vi "Write Pulse Recorder Configuration.vi"(8 "error in (no error)":errorcluster, 10 "Configuration":T1={"Pre-trigger duration"=0.01, "Post-trigger duration"=0.1, "Rate"=1000000.0, "Ranges"=[10.0], "Re-name channels"=[], "Active channels"="0:1", "External clock"=FALSE} {"Rate" format="%#_8pHz"; "Post-trigger duration" format="%#_6ps"; "Pre-trigger duration" format="%#_6ps"; "Ranges" format="%#_6pV"}, 11 "Pulse Recorder in":refnum<class "Pulse Recorder.lvclass">) -> (0 "error out":errorcluster, 3 "Pulse Recorder out":refnum<class "Pulse Recorder.lvclass">)   [LabVIEW 2016, in "Pulse Recorder.lvclass"]
uses:
  Pulse Recorder.lvclass
  C:/github/LabActor/Template Module/Template Module.lvclass
  NHMFL_Core/Libraries/Instruments/Pulse Driver/Pusle Driver Configuration.ctl
  Template Module/Template Module.lvclass/Template Module.ctl
  Template Module/Write Configuration.vi
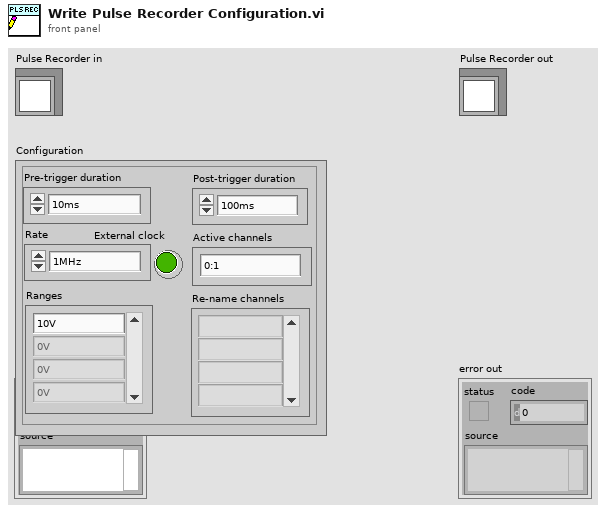
[diagram p1: front panel]
types:
  T1 = typedef "Pusle Driver Configuration.ctl" = cluster{"Pre-trigger duration":dbl, "Post-trigger duration":dbl, "Rate":dbl, "Ranges":dbl[], "Re-name channels":string[], "Active channels":string, "External clock":bool}
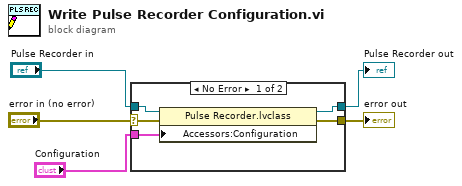
[diagram p0: block diagram]
diagram:
  n1 = case shown="No Error" "error in (no error)" {
    selector: "error in (no error)" -> [w7 w11]
    tunnel: [w6 w11] -> w4
    tunnel: [w8 w12] -> w2
    tunnel: "Pulse Recorder in" -> [w9 w12]
    tunnel: "Configuration" -> [w10 _]
    frame No Error {
      n2 = property class="Pulse Recorder.lvclass"(reference=w9, error in=w7, "Accessors:Configuration"=w10) -> (reference out=w8:refnum<class "Pulse Recorder.lvclass">, error out=w6:errorcluster)
    }
    frame Error {
    }
  }
  "error out" <- w4
  "Pulse Recorder out" <- w2
